vi "Read TDMS Channel-Group Names.vi"(8 "error in":errorcluster, 11 "File Path Control":path) -> (0 "error out":errorcluster, 2 "File-group-channel":T1(array[cluster]))   [LabVIEW 2015]
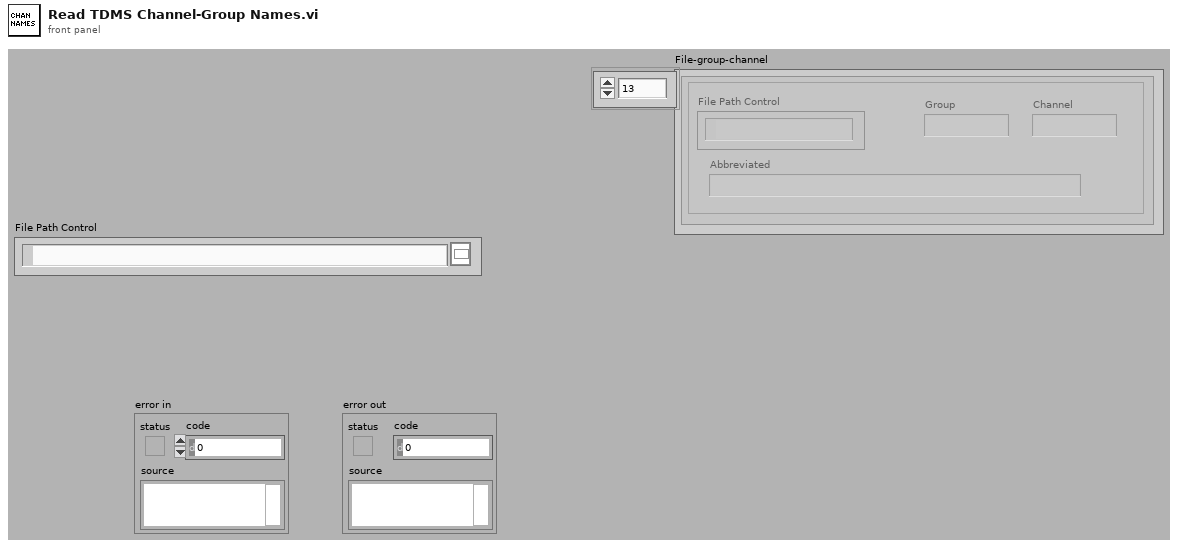
[diagram p1: front panel]
types:
  T1 = cluster{"File Path Control":path, "Group":string, "Channel":string, "Abbreviated":string}[]
  T2 = enum16{"open", "open or create", "create or replace", "create", "open (read-only)"}
  T3 = cluster{"File Path Control":path, string, string, string}
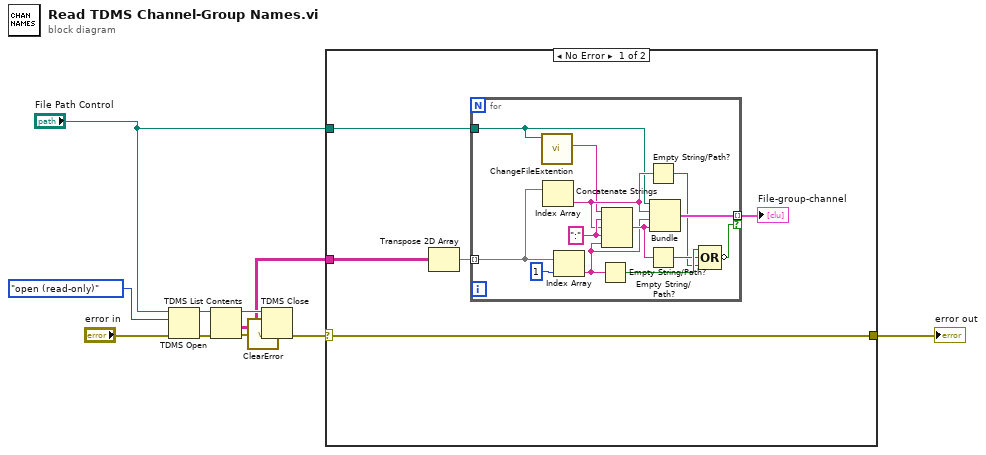
[diagram p0: block diagram]
diagram:
  n1 = TDMS Open(8:"error in", 10:T2."open (read-only)" ("operation (0:open)"), 11:"File Path Control") -> (0:w9:errorcluster, 3:w8:refnum<k34>)  [unwired: 4 in]
  n2 = TDMS List Contents(4:w9, 7:w8) -> (0:w1:errorcluster, 1:w5:string[][], 3:w7:refnum<k34>)  [unwired: 2 out]
  n3 = call <vilib>:"ClearError.vi"("error in (no error)"=w1) -> ("error out"=w6:errorcluster)
  n4 = TDMS Close(8:w6, 11:w7) -> (0:w3:errorcluster)  [unwired: 1 out]
  n5 = case shown="No Error" w3 {
    selector: w3 -> [w12 w30]
    tunnel: w5 -> [w16 _]
    tunnel: "File Path Control" -> [w13 _]
    tunnel: [w12 w30] -> w2
    frame No Error {
      n6 = Transpose 2D Array(2D array=w16) -> (transposed array=w14:string[][])
      n7 = for {
        tunnel: w14 -> [w28] mode=indexing
        tunnel: w13 -> [w18]
        tunnel: [w29] -> w15 mode=indexing if=w20
        w26 = ":"
        n8 = call "ChangeFileExtention.vi"("Path"=w18) -> ("Name before extension"=w17:string)  [unwired: 6 in, 4 out]
        n9 = Index Array(array=w28) -> (element=w24:string)  [unwired: 1 in]
        n10 = Index Array(array=w28, index=1) -> (element=w19:string)
        n11 = Empty String/Path?(string/path=w19) -> (empty?=w23:bool)
        n12 = Concatenate Strings(w17, w26, w24, w26, w19) -> (w25:string)
        n13 = Empty String/Path?(string/path=w24) -> (empty?=w21:bool)
        n14 = Empty String/Path?(string/path=w25) -> (empty?=w22:bool)
        n15 = Bundle("File Path Control"=w18, w24, w19, w25) -> (w29:T3)  [unwired: 1 in]
        n16 = Compound Arithmetic op=OR(w23, w22, w21) -> (invert w20:bool)
      }
      "File-group-channel" <- w15
    }
    frame Error {
    }
  }
  "error out" <- w2
